vi "maintest.vi"() -> ()   [LabVIEW 2015]
uses:
  simulated/simulated.lvclass
  hardware v1/hardware v1.lvclass
  interface/interface.lvclass
panel:
  in  "motor voltage":dbl
  in  "Hardware type":enum16{"simulated", "hardware v1"}(ring)
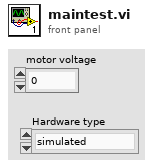
[diagram p1: front panel]
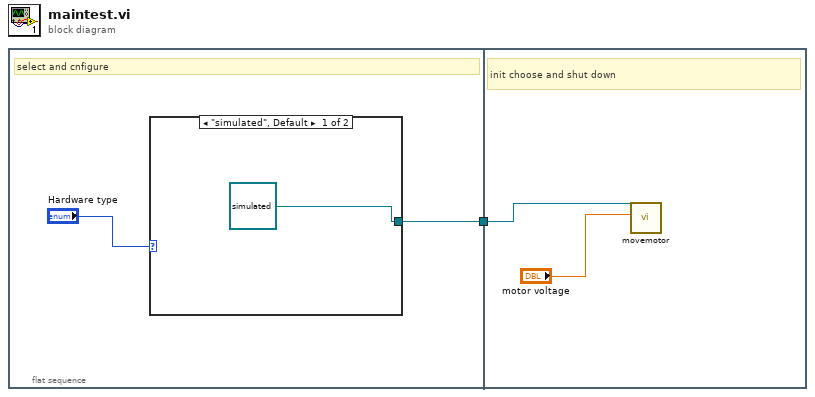
[diagram p0: block diagram]
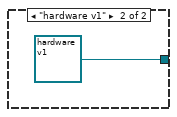
[diagram p2: hidden frame]
diagram:
  n1 = flat-sequence {
    tunnel: [w2] -> w1
    tunnel: w1 -> [w7]
    frame #0 {
      # "select and cnfigure"
      n2 = case shown="\"simulated\", Default" "Hardware type" {
        tunnel: [refnum<class "simulated.lvclass"> refnum ("simulated in") refnum<class "hardware v1.lvclass"> refnum ("hardware v1 in")] -> w2
        frame "simulated", Default {
        }
        frame "hardware v1" {
        }
      }
    }
    frame #1 {
      # "init choose and shut down"
      n3 = call-dynamic "movemotor.vi"("motor voltage"="motor voltage", "interface in"=w7) -> ()  [unwired: 8 in, 2 out]
    }
  }
